vi "NI-XNET Create CAN Cluster.vi"(8 "error in":errorcluster, 10 "CAN Cluster":T1={"Baud Rate"=125000, "Comment"="", "Name"=""}, 11 "database in":refnum<k21>) -> (0 "error out":errorcluster, 3 "cluster out":refnum<k21>)   [LabVIEW 2023, in "NEO480HTA.lvlib"]
uses:
  Devices/NEO480HTA.lvlib
  <vilib>/xnet/xnet.llb/XNET Database Create (Cluster).vi
  <resource>/objmgr/xnet.rc
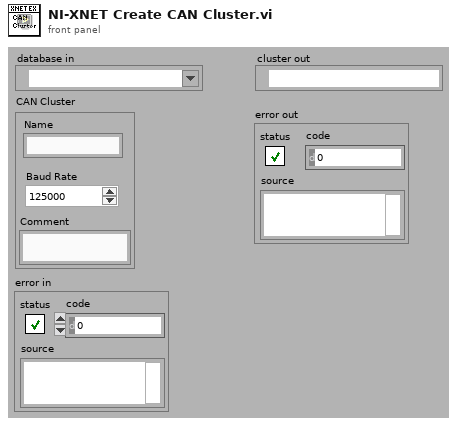
[diagram p1: front panel]
types:
  T1 = cluster{"Baud Rate":u32, "Comment":string, "Name":string}
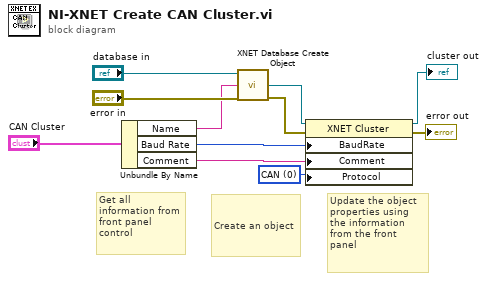
[diagram p0: block diagram]
diagram:
  w11 = u32 0 items=["CAN", "FlexRay"] ("Protocol")
  # "Update the object properties using the information from the front panel"
  # "Create an object"
  # "Get all information from front panel control"
  n1 = Unbundle By Name("CAN Cluster") -> ("Name"=w6:string, "Baud Rate"=w7:u32, "Comment"=w8:string)
  n2 = call-poly <vilib>:"XNET Database Create Object.vi"("database in"="database in", "cluster name"=w6, "error in (no error)"="error in") -> ("cluster out"=w1:refnum<k21>, "error out"=w5:errorcluster)  [unwired: 10 in, 1 out]
  n3 = property class="XNET Cluster"(reference=w1, error in=w5, "BaudRate"=w7, "Comment"=w8, "Protocol"=w11) -> (reference out=→"cluster out":refnum<k21>, error out=→"error out":errorcluster)
